vi "Init from Strings.vi"(7 "Index":string, 8 "Error In":errorcluster, 9 "Values":string[](array[string]), 10 "Keys":string[](array[string]), 11 "reference in":refnum<class "OD Entry.lvclass">) -> (0 "Error Out":errorcluster, 3 "reference out":refnum<class "OD Entry.lvclass">)   [LabVIEW 2024, in "EDS.lvlib" / "OD Entry.lvclass"]
doc: "Indices in the EDS are always in hex format without the pre 0x"
uses:
  OD Entry.lvclass
  OD Entry.lvclass/OD Entry.ctl
  Object Type.ctl
  EDS.lvlib
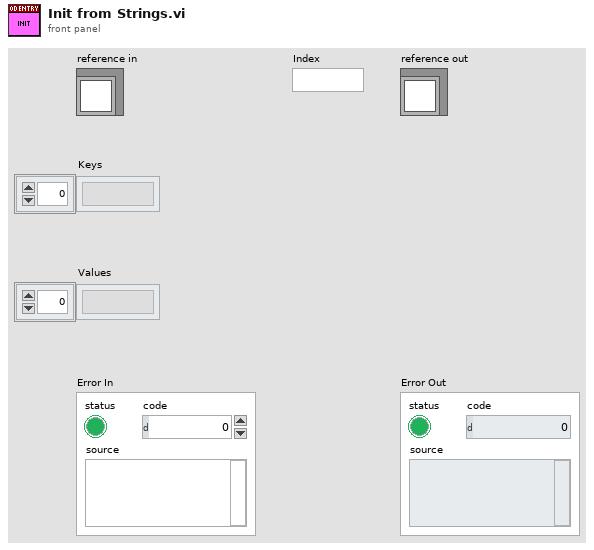
[diagram p1: front panel]
types:
  T1 = typedef "EDS.lvlib/OD Entry.lvclass/ObjectAttributes.ctl" = cluster{"Index":u16, "ParameterName":string, "Denotation":string, "ObjectType":T2, "DataType":T3, "AccessType":T4, "DefaultValue":string, "LowLimit":string, "HighLimit":string, "ObjFlags":u32, "CompactSubObj":u8, "PDOMapping":bool, "Count":u8, "ObjExtend":u8, "PDOtype":T5, "Label":string, "Description":string, "Sub-Entries":map{u16, refnum<class "OD Sub-Entry.lvclass">}}
  T2 = typedef "EDS.lvlib/Object Type.ctl" = i16
  T3 = typedef "EDS.lvlib/Data Type.ctl" = enum16{"UNKNOWN", "BOOLEAN", "INTEGER8", "INTEGER16", "INTEGER32", "UNSIGNED8", "UNSIGNED16", "UNSIGNED32", "REAL32", "VISIBLE_STRING", "OCTET_STRING", "UNICODE_STRING", "TIME_OF_DAY", "TIME_DIFFERENCE", "RESERVED1", "DOMAIN", "INTEGER24", "REAL64", "INTEGER40", "INTEGER48", "INTEGER56", "INTEGER64", "UNSIGNED24", "RESERVED2", "UNSIGNED40", "UNSIGNED48", "UNSIGNED56", "UNSIGNED64", "RESERVED3", "RESERVED4", "RESERVED5", "RESERVED6", "PDO_COMMUNICATION_PARAMETER", "PDO_MAPPING", "SDO_PARAMETER", "IDENTITY", "RESERVED7"}
  T4 = typedef "EDS.lvlib/Access Type.ctl" = enum16{"rw", "ro", "wo", "rwr", "rww", "const", "UNKNOWN"}
  T5 = typedef "EDS.lvlib/PDO Mapping Type.ctl" = enum16{"NO", "OPTIONAL", "RPDO", "TPDO", "DEFAULT"}
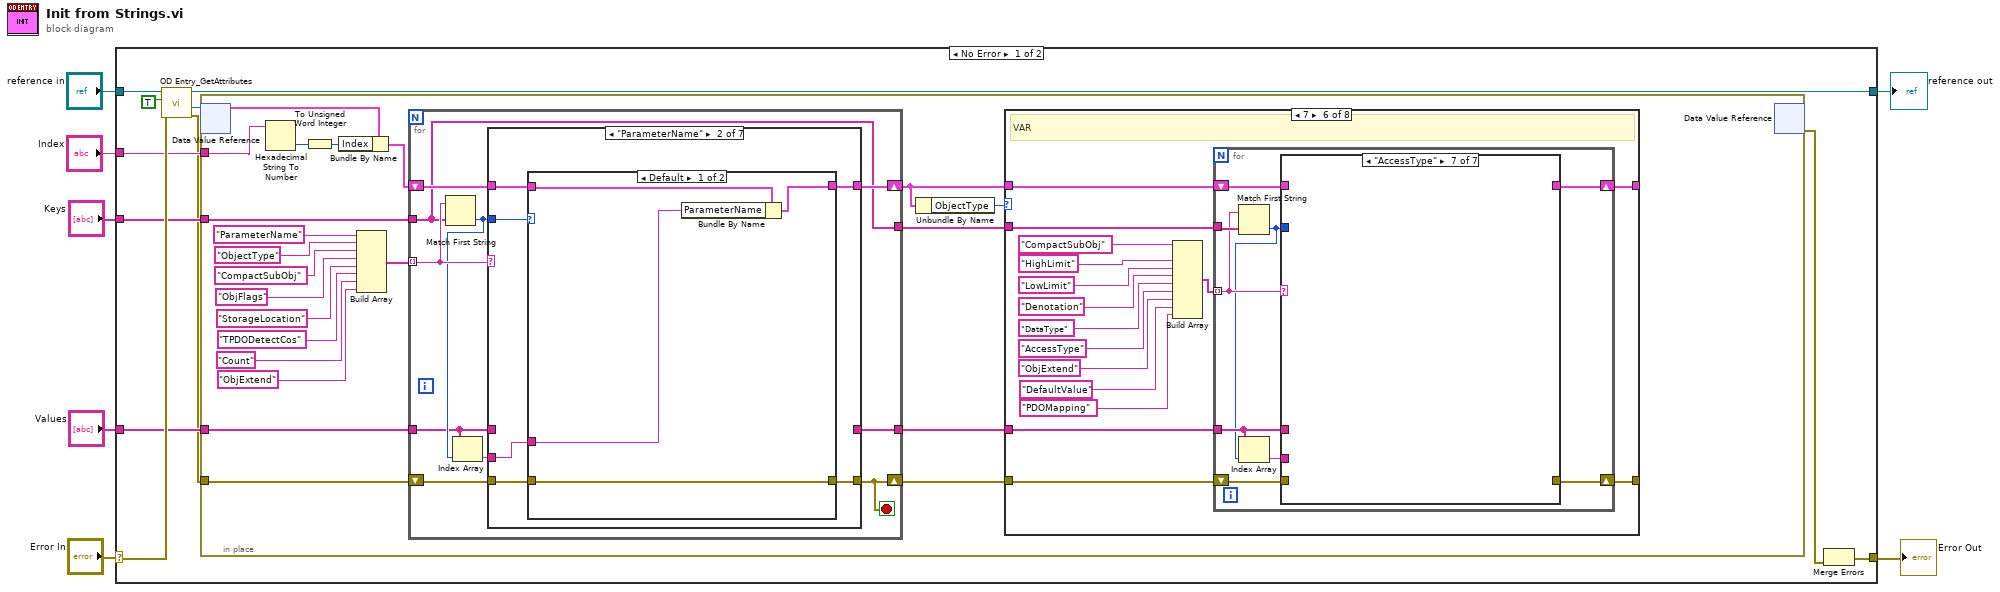
[diagram p0: block diagram]
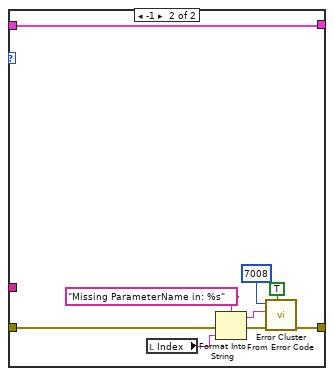
[diagram p3: hidden frame]
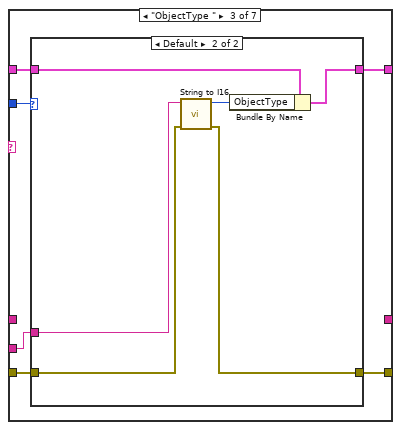
[diagram p4: hidden frame]
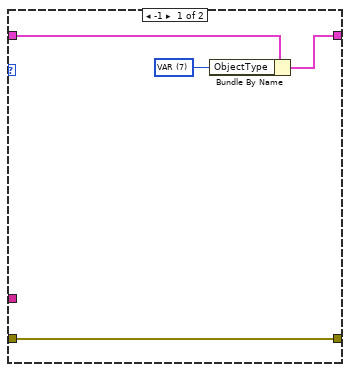
[diagram p5: hidden frame]
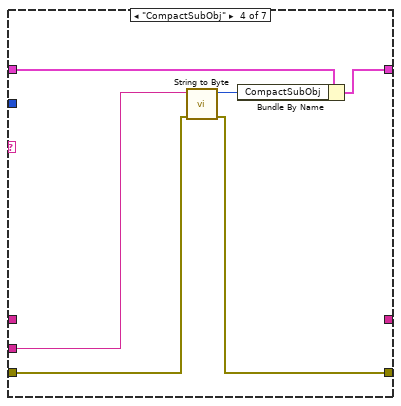
[diagram p6: hidden frame]
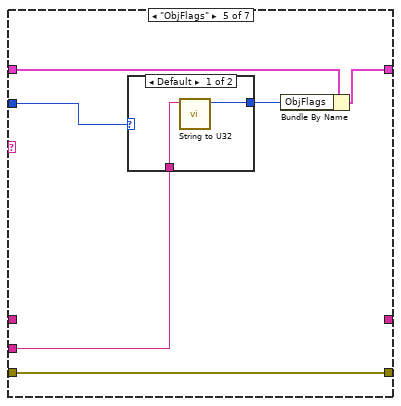
[diagram p7: hidden frame]
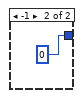
[diagram p8: hidden frame]
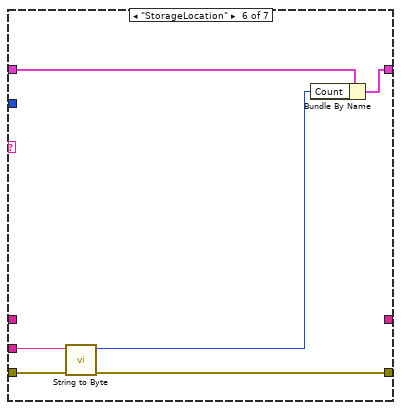
[diagram p9: hidden frame]
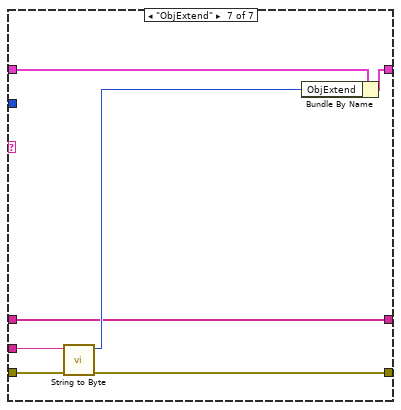
[diagram p10: hidden frame]
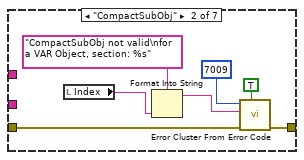
[diagram p17: hidden frame]
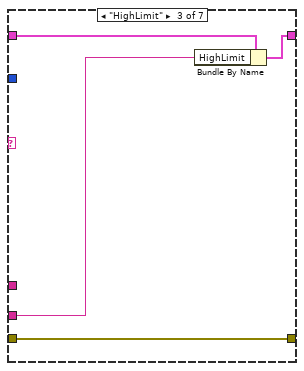
[diagram p18: hidden frame]
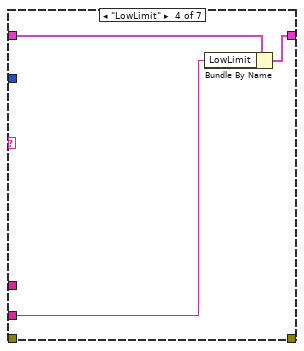
[diagram p19: hidden frame]
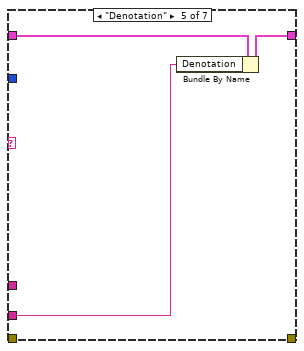
[diagram p20: hidden frame]
diagram:
  n1 = case shown="No Error" "Error In" {
    selector: "Error In" -> [w16 w180]
    tunnel: [w12 w180] -> w6
    tunnel: [w17 w179] -> w4
    tunnel: "reference in" -> [w18 w179]
    tunnel: "Index" -> [w11 _]
    tunnel: "Keys" -> [w10 _]
    tunnel: "Values" -> [w9 _]
    frame No Error {
      n2 = call "OD Entry_GetAttributes.vi"("Error In"=w16, "OnlyGetDvrReference(False)"=TRUE, "reference in"=w18) -> ("Error Out"=w8:errorcluster, "DataRef"=w13:refnum<data-value>, "reference out"=w17:refnum<class "OD Entry.lvclass">)  [unwired: 5 in, 1 out]
      n3 = in-place {
        in-place-border: w11 -> [w35]
        in-place-border: w10 -> [w37]
        in-place-border: w9 -> [w36]
        in-place-border: w8 -> [w38]
        n4 = in-place-dvr #1(w13) -> (w25:T1)  [unwired: 1 out]
        n5 = Hexadecimal String To Number(string=w35) -> (number=w40:u32)  [unwired: 2 in, 1 out]
        n6 = To Unsigned Word Integer(number=w40) -> (unsigned 16bit integer=w39:u16)
        n7 = Bundle By Name(cluster=w25, "Index"=w39) -> (w24:T1)
        n8 = Build Array("ParameterName", "ObjectType", "CompactSubObj", "ObjFlags", "StorageLocation", "TPDODetectCos", "Count", "ObjExtend") -> (w32:string[])
        n9 = for {
          tunnel: w36 -> [w42]
          tunnel: w37 -> [w43]
          shift-right: [w48] -> w22
          shift-left: w24 -> [w49]
          tunnel: w32 -> [w47] mode=indexing
          shift-right: [w44] -> w20
          shift-left: w38 -> [w50]
          tunnel: [w43] -> w21
          tunnel: [w41] -> w19
          stop <- w44 stop-if-true
          n10 = Match First String(2:w43, 3:w47) -> (0:w46:i32)  [unwired: 1 out]
          n11 = Index Array(array=w42, index=w46) -> (element=w45:string)
          n12 = case shown="\"ParameterName\"" w47 {
            tunnel: w50 -> [w51 w58 w72 w89 w96 w106 w113]
            tunnel: w49 -> [w52 w55 w77 w93 w99 w108 w115]
            tunnel: [w52 w54 w76 w92 w98 w107 w114] -> w48
            tunnel: w46 -> [_ w56 w75 _ w94 _ _]
            tunnel: [w51 w57 w73 w88 w96 w103 w110] -> w44
            tunnel: w45 -> [_ w53 w74 w91 w97 w105 w112]
            tunnel: w42 -> [_ _ _ _ _ _ w109]
            tunnel: [_ _ _ _ _ _ w109] -> w41
            frame Default {
            }
            frame "ParameterName" {
              # "Parameter name is mandatory"
              n13 = case shown="Default" w56 {
                tunnel: w58 -> [w62 w66]
                tunnel: [w62 w64] -> w57
                tunnel: w55 -> [w61 w63]
                tunnel: [w60 w63] -> w54
                tunnel: w53 -> [w59 _]
                frame Default {
                  n14 = Bundle By Name(cluster=w61, "ParameterName"=w59) -> (w60:T1)
                }
                frame -1 {
                  n15 = local read "Index"() -> (w65:string)
                  n16 = Format Into String(format string="Missing ParameterName in: %s", error in=w66, w65) -> (resulting string=w70:string, error out=w71:errorcluster)  [unwired: 1 in]
                  n17 = call <vilib>:"Error Cluster From Error Code.vi"("show call chain? (False)"=TRUE, "error in (no error)"=w71, "error message (\"\")"=w70, "error code (0)"=7008) -> ("error out"=w64:errorcluster)  [unwired: 5 in]
                }
              }
            }
            frame "ObjectType " {
              n18 = case shown="Default" w75 {
                tunnel: w77 -> [w81 w87]
                tunnel: [w80 w86] -> w76
                tunnel: w74 -> [_ w84]
                tunnel: w72 -> [w78 w83]
                tunnel: [w78 w82] -> w73
                frame -1 {
                  w79 = T2 7 items=["UNKNOWN"=-1, "NULL"=0, "DOMAIN"=2, "DEFTYPE"=5, "DEFSTRUCT"=6, "VAR"=7, "ARRAY"=8, "RECORD"=9] ("ObjectType")
                  n19 = Bundle By Name(cluster=w81, "ObjectType"=w79) -> (w80:T1)
                }
                frame Default {
                  n20 = call "String to I16.vi"("error in"=w83, "String"=w84) -> ("error out"=w82:errorcluster, "I16"=w85:i16)  [unwired: 8 in]
                  n21 = Bundle By Name(cluster=w87, "ObjectType"=w85) -> (w86:T1)
                }
              }
            }
            frame "CompactSubObj" {
              n22 = call "String to Byte.vi"("error in"=w89, "String"=w91) -> ("error out"=w88:errorcluster, "Byte"=w90:u8)  [unwired: 8 in]
              n23 = Bundle By Name(cluster=w93, "CompactSubObj"=w90) -> (w92:T1)
            }
            frame "ObjFlags" {
              n24 = case shown="Default" w94 {
                tunnel: w97 -> [w101 _]
                tunnel: [w100 u32 0 ("U32")] -> w95
                frame Default {
                  n25 = call "String to U32.vi"("String"=w101) -> ("U32"=w100:u32)  [unwired: 10 in]
                }
                frame -1 {
                }
              }
              n26 = Bundle By Name(cluster=w99, "ObjFlags"=w95) -> (w98:T1)
            }
            frame "StorageLocation" {
              n27 = call "String to Byte.vi"("error in"=w106, "String"=w105) -> ("error out"=w103:errorcluster, "Byte"=w104:u8)  [unwired: 8 in]
              n28 = Bundle By Name(cluster=w108, "Count"=w104) -> (w107:T1)
            }
            frame "ObjExtend" {
              n29 = call "String to Byte.vi"("error in"=w113, "String"=w112) -> ("error out"=w110:errorcluster, "Byte"=w111:u8)  [unwired: 8 in]
              n30 = Bundle By Name(cluster=w115, "ObjExtend"=w111) -> (w114:T1)
            }
          }
        }
        n31 = Unbundle By Name(w22) -> ("ObjectType"=w23:T2)
        n32 = case shown="7" w23 {
          tunnel: w22 -> [_ _ _ _ _ w118 _ _]
          tunnel: w21 -> [_ _ _ _ _ w121 _ _]
          tunnel: w20 -> [_ _ _ _ _ w120 _ _]
          tunnel: [_ _ _ _ _ w119 _ _] -> _
          tunnel: [_ _ _ _ _ w117 _ _] -> _
          tunnel: w19 -> [_ _ _ _ _ w116 _ _]
          frame -1 {
            # "UNKNOWN"
          }
          frame 0 {
            # "NULL"
          }
          frame 2 {
            # "DOMAIN"
          }
          frame 5 {
            # "DEFTYPE"
          }
          frame 6 {
            # "DEFSTRUCT"
          }
          frame 7 {
            # "VAR"
            n33 = Build Array("CompactSubObj", "HighLimit", "LowLimit", "Denotation", "DataType", "AccessType", "ObjExtend", "DefaultValue", "PDOMapping") -> (w124:string[])  [unwired: 1 in]
            n34 = for {
              tunnel: w124 -> [w139] mode=indexing
              tunnel: w121 -> [w140]
              shift-right: [w137] -> w119
              shift-left: w120 -> [w138]
              shift-right: [w135] -> w117
              shift-left: w118 -> [w136]
              tunnel: w116 -> [w134]
              n35 = Match First String(2:w140, 3:w139) -> (0:w133:i32)  [unwired: 1 out]
              n36 = Index Array(array=w134, index=w133) -> (element=w132:string)
              n37 = case shown="\"AccessType\"" w139 {
                tunnel: w133 -> [_ _ _ _ _ w164 _]
                tunnel: w138 -> [_ w147 w151 _ _ w163 _]
                tunnel: [_ w141 w151 _ _ w162 _] -> w137
                tunnel: w136 -> [_ _ w150 w154 w157 w159 _]
                tunnel: [_ _ w149 w153 w156 w158 _] -> w135
                tunnel: w134 -> [_ _ _ _ _ _ _]
                tunnel: w132 -> [_ _ w148 w152 w155 w160 _]
                frame Default {
                }
                frame "CompactSubObj" {
                  n38 = local read "Index"() -> (w143:string)
                  n39 = Format Into String(format string="CompactSubObj not valid\nfor a VAR Object, section: %s", w143) -> (resulting string=w142:string)  [unwired: 2 in, 1 out]
                  n40 = call <vilib>:"Error Cluster From Error Code.vi"("show call chain? (False)"=TRUE, "error in (no error)"=w147, "error message (\"\")"=w142, "error code (0)"=7009) -> ("error out"=w141:errorcluster)  [unwired: 5 in]
                }
                frame "HighLimit" {
                  n41 = Bundle By Name(cluster=w150, "HighLimit"=w148) -> (w149:T1)
                }
                frame "LowLimit" {
                  n42 = Bundle By Name(cluster=w154, "LowLimit"=w152) -> (w153:T1)
                }
                frame "Denotation" {
                  n43 = Bundle By Name(cluster=w157, "Denotation"=w155) -> (w156:T1)
                }
                frame "DataType" {
                  n44 = Less Or Equal To 0?(x=w164) -> (x <= 0?=w161:bool)
                  n45 = case "DataType missing?" shown="True" w161 {
                    tunnel: w163 -> [w166 w176]
                    tunnel: [w165 w173] -> w162
                    tunnel: w160 -> [w167 _]
                    tunnel: w159 -> [w170 w171]
                    tunnel: [w169 w171] -> w158
                    frame False {
                      n46 = call "String to I16.vi"("error in"=w166, "String"=w167) -> ("error out"=w165:errorcluster, "I16"=w168:i16)  [unwired: 8 in]
                      n47 = Bundle By Name(cluster=w170, "DataType"=w168) -> (w169:T1)
                    }
                    frame True {
                      n48 = local read "Index"() -> (w177:string)
                      n49 = Format Into String(format string="Missing required field \nDataType on %s", w177) -> (resulting string=w175:string)  [unwired: 2 in, 1 out]
                      n50 = call <vilib>:"Error Cluster From Error Code.vi"("show call chain? (False)"=TRUE, "error in (no error)"=w176, "error message (\"\")"=w175, "error code (0)"=7010) -> ("error out"=w173:errorcluster)  [unwired: 5 in]
                    }
                  }
                }
                frame "AccessType" {
                }
              }
            }
          }
          frame 8 {
            # "ARRAY"
          }
          frame 9 {
            # "RECORD"
          }
        }
        n51 = in-place-dvr #1() -> (w14:errorcluster)  [unwired: 1 in, 1 out]
      }
      n52 = Merge Errors(w14) -> (w12:errorcluster)  [unwired: 1 in]
    }
    frame Error {
    }
  }
  "Error Out" <- w6
  "reference out" <- w4
